vi "Create PUBLISH Packet.vi"(4 "RETAIN":bool, 5 "PUBLISH type":refnum<class "PUBLISH.lvclass">, 6 "QoS":T1, 7 "DUP (Re-delivery attempt)":bool, 8 "error in (no error)":errorcluster, 9 "Packet ID (empty: generate new)":u16 format="%04x", 10 "Payload":u8[](array[numeric]) format="%08b", 11 "Topic Name":string) -> (0 "error out":errorcluster, 1 "Packet ID":u16 format="%04x", 3 "PUBLISH":refnum<class "PUBLISH.lvclass">)   [LabVIEW 2013, in "PUBLISH.lvclass"]
uses:
  PUBLISH.lvclass
  ControlPacket/QualityOfService -- enum.ctl
  ControlPacket/ControlPacket.lvclass/ControlPacket.ctl
  ControlPacket/ControlPacket.lvclass
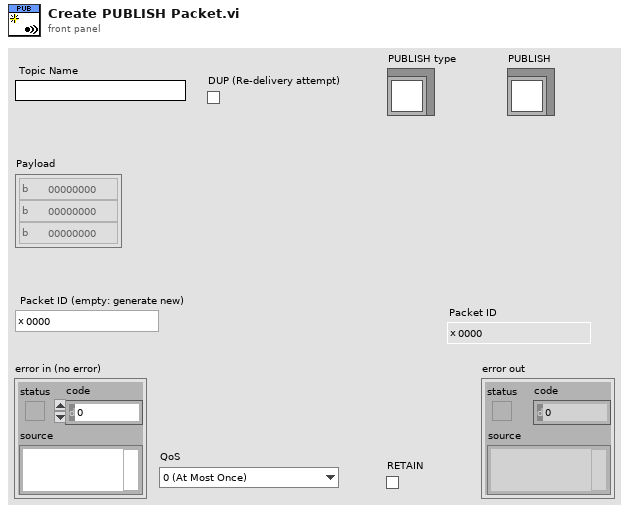
[diagram p1: front panel]
types:
  T1 = typedef "ControlPacket.lvclass/QualityOfService -- enum.ctl" = enum16{"0 (At Most Once)", "1 (At Least Once)", "2 (Exactly Once)"}
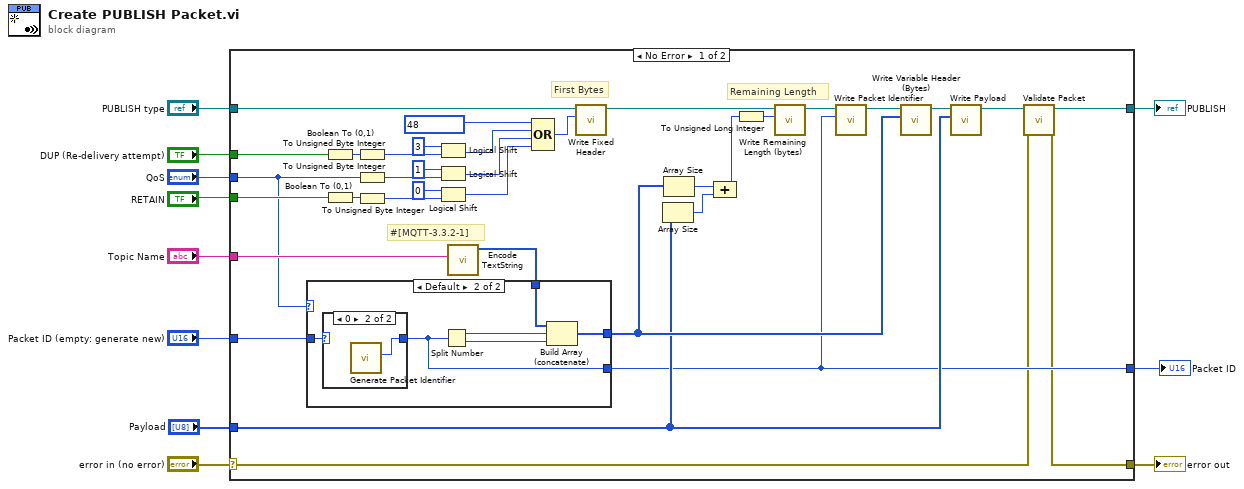
[diagram p0: block diagram]
diagram:
  n1 = case shown="No Error" "error in (no error)" {
    selector: "error in (no error)" -> [w14 w57]
    tunnel: [w13 w57] -> w10
    tunnel: [w15 w56] -> w8
    tunnel: "PUBLISH type" -> [w31 w56]
    tunnel: "DUP (Re-delivery attempt)" -> [w33 _]
    tunnel: "RETAIN" -> [w46 _]
    tunnel: "QoS" -> [w12 _]
    tunnel: "Topic Name" -> [w32 _]
    tunnel: "Packet ID (empty: generate new)" -> [w18 _]
    tunnel: "Payload" -> [w24 _]
    tunnel: [w17 _] -> w1
    frame No Error {
      # "#[MQTT-3.3.2-1]"
      # "Remaining Length"
      # "First Bytes"
      n2 = Boolean To (0,1)(Boolean=w33) -> (0, 1=w42:i16)
      n3 = Boolean To (0,1)(Boolean=w46) -> (0, 1=w41:i16)
      n4 = To Unsigned Byte Integer(number=w42) -> (unsigned 8bit integer=w43:u8)
      n5 = To Unsigned Byte Integer(number=w12) -> (unsigned 8bit integer=w40:u8)
      n6 = To Unsigned Byte Integer(number=w41) -> (unsigned 8bit integer=w39:u8)
      n7 = Logical Shift(y=i16 3, x=w43) -> (x << y=w44:u8)
      n8 = Logical Shift(y=i16 1, x=w40) -> (x << y=w38:u8)
      n9 = Logical Shift(y=i16 0, x=w39) -> (x << y=w37:u8)
      n10 = call "Encode TextString.vi"("Text String"=w32) -> ("Length-Prefixed Field"=w26:u8[])  [unwired: 10 in]
      n11 = case shown="Default" w12 {
        tunnel: w26 -> [w47 w53]
        tunnel: [w47 w50] -> w25
        tunnel: w18 -> [_ w49]
        tunnel: [_ w48] -> w17
        frame "0 (At Most Once)" {
          # "#[MQTT-2.3.1-5]"
        }
        frame Default {
          n12 = case shown="0" w49 {
            selector: w49 -> [w54 _]
            tunnel: [w54 w55] -> w48
            frame Default {
            }
            frame 0 {
              n13 = call "Generate Packet Identifier.vi"() -> ("Packet Identifier"=w55:u16)  [unwired: 11 in]
            }
          }
          n14 = Split Number(x=w48) -> (hi(x)=w52:u8, lo(x)=w51:u8)
          n15 = Build Array (concatenate)(w53, w52, w51) -> (w50:u8[])
        }
      }
      n16 = Compound Arithmetic op=OR(u8 48, w44, w38, w37) -> (w30:u8)
      n17 = call "Write Fixed Header.vi"("Fixed Header"=w30, "ControlPacket in"=w31) -> ("ControlPacket out"=w28:refnum<class "PUBLISH.lvclass">)  [unwired: 9 in]
      n18 = Array Size(array=w24) -> (size(s)=w22:i32)
      n19 = Array Size(array=w25) -> (size(s)=w23:i32)
      n20 = Compound Arithmetic op=ADD(w23, w22) -> (w21:i32)
      n21 = To Unsigned Long Integer(number=w21) -> (unsigned 32bit integer=w29:u32)
      n22 = call "Write Remaining Length (bytes).vi"("Remaining Length (bytes)"=w29, "ControlPacket in"=w28) -> ("ControlPacket out"=w20:refnum<class "PUBLISH.lvclass">)  [unwired: 9 in]
      n23 = call "Write Packet Identifier.vi"("Packet Identifier"=w17, "ControlPacket in"=w20) -> ("ControlPacket out"=w19:refnum<class "PUBLISH.lvclass">)  [unwired: 9 in]
      n24 = call "Write Variable Header (Bytes).vi"("Variable Header (Bytes)"=w25, "ControlPacket in"=w19) -> ("ControlPacket out"=w27:refnum<class "PUBLISH.lvclass">)  [unwired: 9 in]
      n25 = call "Write Payload.vi"("Payload"=w24, "ControlPacket in"=w27) -> ("ControlPacket out"=w16:refnum<class "PUBLISH.lvclass">)  [unwired: 9 in]
      n26 = call "Validate Packet.vi"("error in (no error)"=w14, "ControlPacket in"=w16) -> ("error out"=w13:errorcluster, "ControlPacket out"=w15:refnum<class "PUBLISH.lvclass">)  [unwired: 8 in]
    }
    frame Error {
    }
  }
  "error out" <- w10
  "PUBLISH" <- w8
  "Packet ID" <- w1
